vi "双向画图.vi"(1 "电流数据":dbl[](array[numeric]), 2 "电压改变量":dbl, 3 "反向扫描电压(V)":dbl min=0.0 max=40.0 step=0.1, 4 "正向扫描电压(V)":dbl min=0.0 max=40.0 step=0.1) -> (0 "XY图":picture)   [LabVIEW 2019]
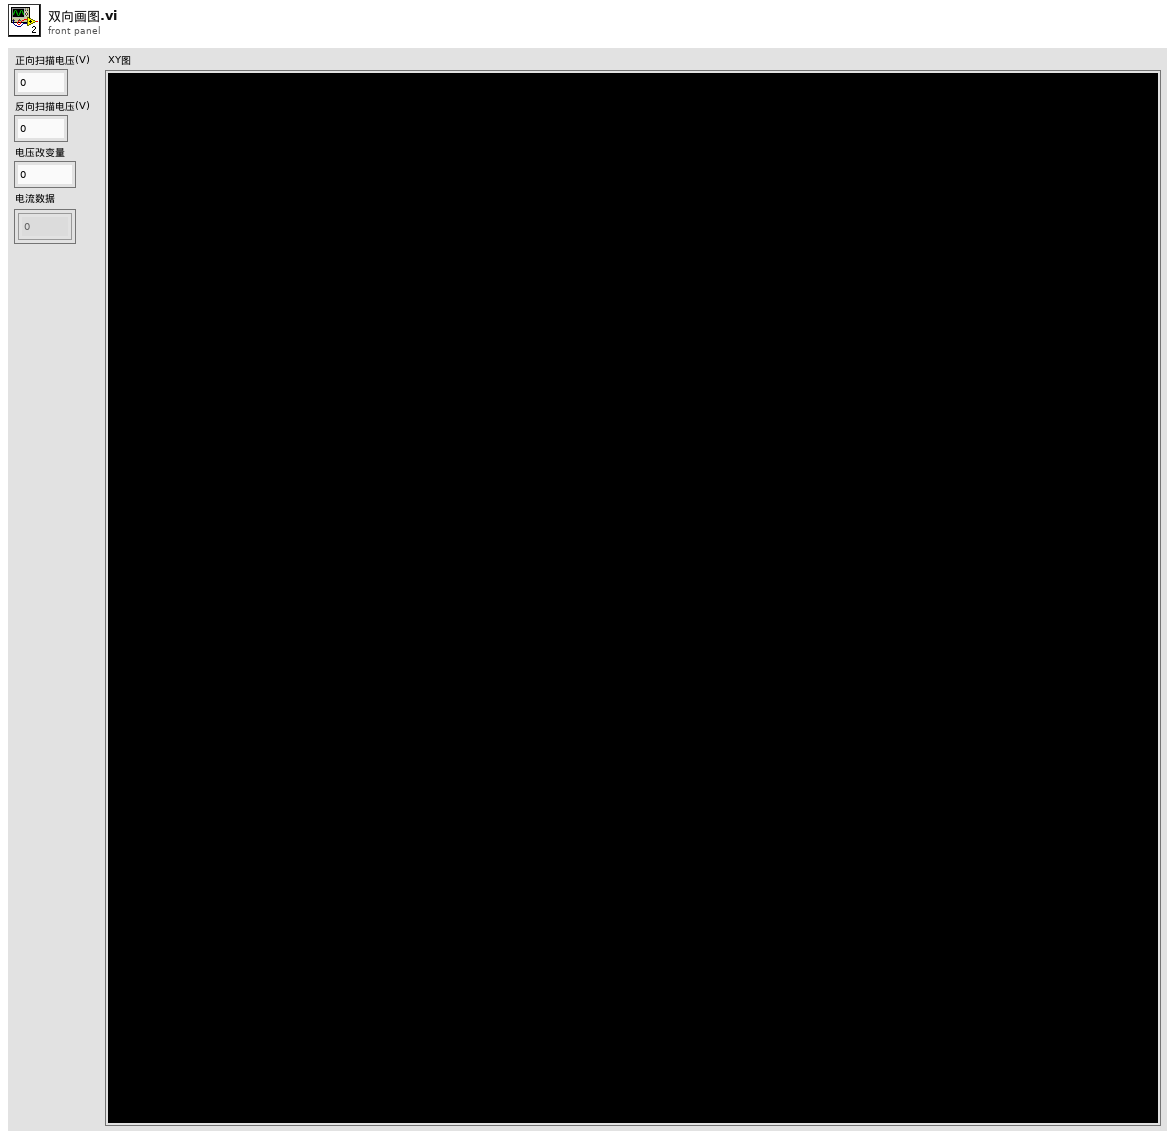
[diagram p1: front panel]
types:
  T1 = enum8{"Decimal", "Scientific", "Engineering", "Binary", "Octal", "Hex"}
  T2 = cluster{dbl, dbl, "x log?":bool, "x precision":u8, "x format":enum8{"Decimal", "Scientific", "Engineering", "Binary", "Octal", "Hex"}, dbl, dbl, "y log?":bool, "y precision":u8, "y format":enum8{"Decimal", "Scientific", "Engineering", "Binary", "Octal", "Hex"}}
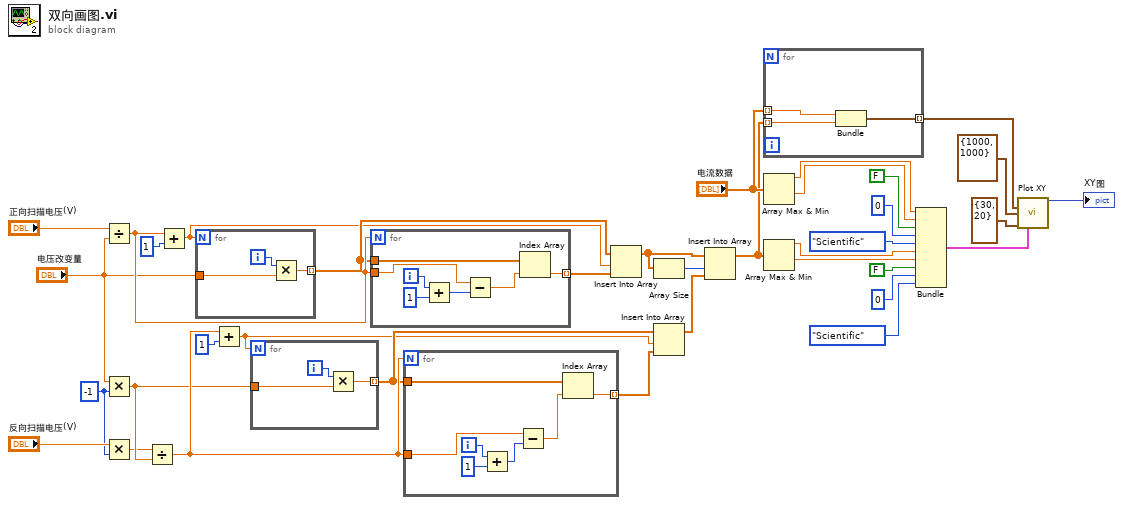
[diagram p0: block diagram]
diagram:
  w2 = -1
  n1 = Divide(x="正向扫描电压(V)", y="电压改变量") -> (x/y=w19:dbl)
  n2 = Multiply(x="电压改变量", y=w2) -> (x*y=w8:dbl)
  n3 = Multiply(x="反向扫描电压(V)", y=w2) -> (x*y=w3:dbl)
  n4 = Divide(x=w3, y=w8) -> (x/y=w13:dbl)
  n5 = Add(x=w19, y=1) -> (x+y=w16:dbl)
  n6 = for {
    N: w16 -> [_]
    tunnel: "电压改变量" -> [w39]
    tunnel: [w38] -> w18 mode=indexing
    i -> [w37]
    n7 = Multiply(x=w37, y=w39) -> (x*y=w38:dbl)
  }
  n8 = Add(x=w13, y=1) -> (x+y=w10:dbl)
  n9 = for {
    N: w10 -> [_]
    tunnel: w8 -> [w42]
    tunnel: [w41] -> w12 mode=indexing
    i -> [w40]
    n10 = Multiply(x=w40, y=w42) -> (x*y=w41:dbl)
  }
  n11 = for {
    N: w19 -> [_]
    tunnel: w18 -> [w49]
    tunnel: w19 -> [w48]
    tunnel: [w46] -> w17 mode=indexing
    i -> [w45]
    n12 = Add(x=w45, y=1) -> (x+y=w43:i32)
    n13 = Subtract(x=w48, y=w43) -> (x-y=w47:dbl)
    n14 = Index Array(array=w49, index=w47) -> (element=w46:dbl)
  }
  n15 = for {
    N: w13 -> [_]
    tunnel: w12 -> [w56]
    tunnel: w13 -> [w55]
    tunnel: [w53] -> w11 mode=indexing
    i -> [w52]
    n16 = Add(x=w52, y=1) -> (x+y=w50:i32)
    n17 = Subtract(x=w55, y=w50) -> (x-y=w54:dbl)
    n18 = Index Array(array=w56, index=w54) -> (element=w53:dbl)
  }
  n19 = Insert Into Array(array=w18, index=w16, new element=w17) -> (w6:dbl[])
  n20 = Array Size(array=w6) -> (size(s)=w5:i32)
  n21 = Insert Into Array(array=w12, index=w10, new element=w11) -> (w7:dbl[])
  n22 = Insert Into Array(array=w6, index=w5, new element=w7) -> (w1:dbl[])
  n23 = for {
    tunnel: [w59] -> w36 mode=indexing
    tunnel: "电流数据" -> [w58] mode=indexing
    tunnel: w1 -> [w57] mode=indexing
    n24 = Bundle("数值"=w58, w57) -> (w59:cluster{"数值":dbl, dbl})  [unwired: 1 in]
  }
  n25 = Array Max & Min(array="电流数据") -> (max value=w21:dbl, min value=w20:dbl)  [unwired: 2 out]
  n26 = Array Max & Min(array=w1) -> (max value=w24:dbl, min value=w23:dbl)  [unwired: 2 out]
  n27 = Bundle(w21, w20, "x log?"=FALSE, "x precision"=u8 0, "x format"=T1."Scientific", w24, w23, "y log?"=FALSE, "y precision"=u8 0, "y format"=T1."Scientific") -> (w28:T2)  [unwired: 1 in]
  n28 = call <vilib>:"Plot XY.vi"("data"=w36, "dimensions (w,h)"=cluster{"width":i16, "height":i16} {"width"=1000, "height"=1000}, "top left point(0, 0)"=cluster{"x":i16, "y":i16} {"x"=30, "y"=20}, "cartesian axis attributes"=w28) -> ("new picture"=→"XY图":picture)  [unwired: 11 in]
